vi "min data out.vi"(6 "Numeric":i32, 8 "error in (no error)":errorcluster, 9 "out time":string[](array[string]), 10 "in time":string[](array[string]), 11 "Count in":string[](array[string])) -> (0 "error out":errorcluster, 2 "string min":string[](array[string]), 3 "duration":dbl[](array[numeric]), 5 "COUNT OF ARRAY":dbl, 7 "DURATION SUM OF ARRAY":dbl)   [LabVIEW 2017]
panel:
  out "last count in min":dbl[][](array[numeric])
  out "sum":dbl
  out "Array 3":dbl[][](array[numeric])
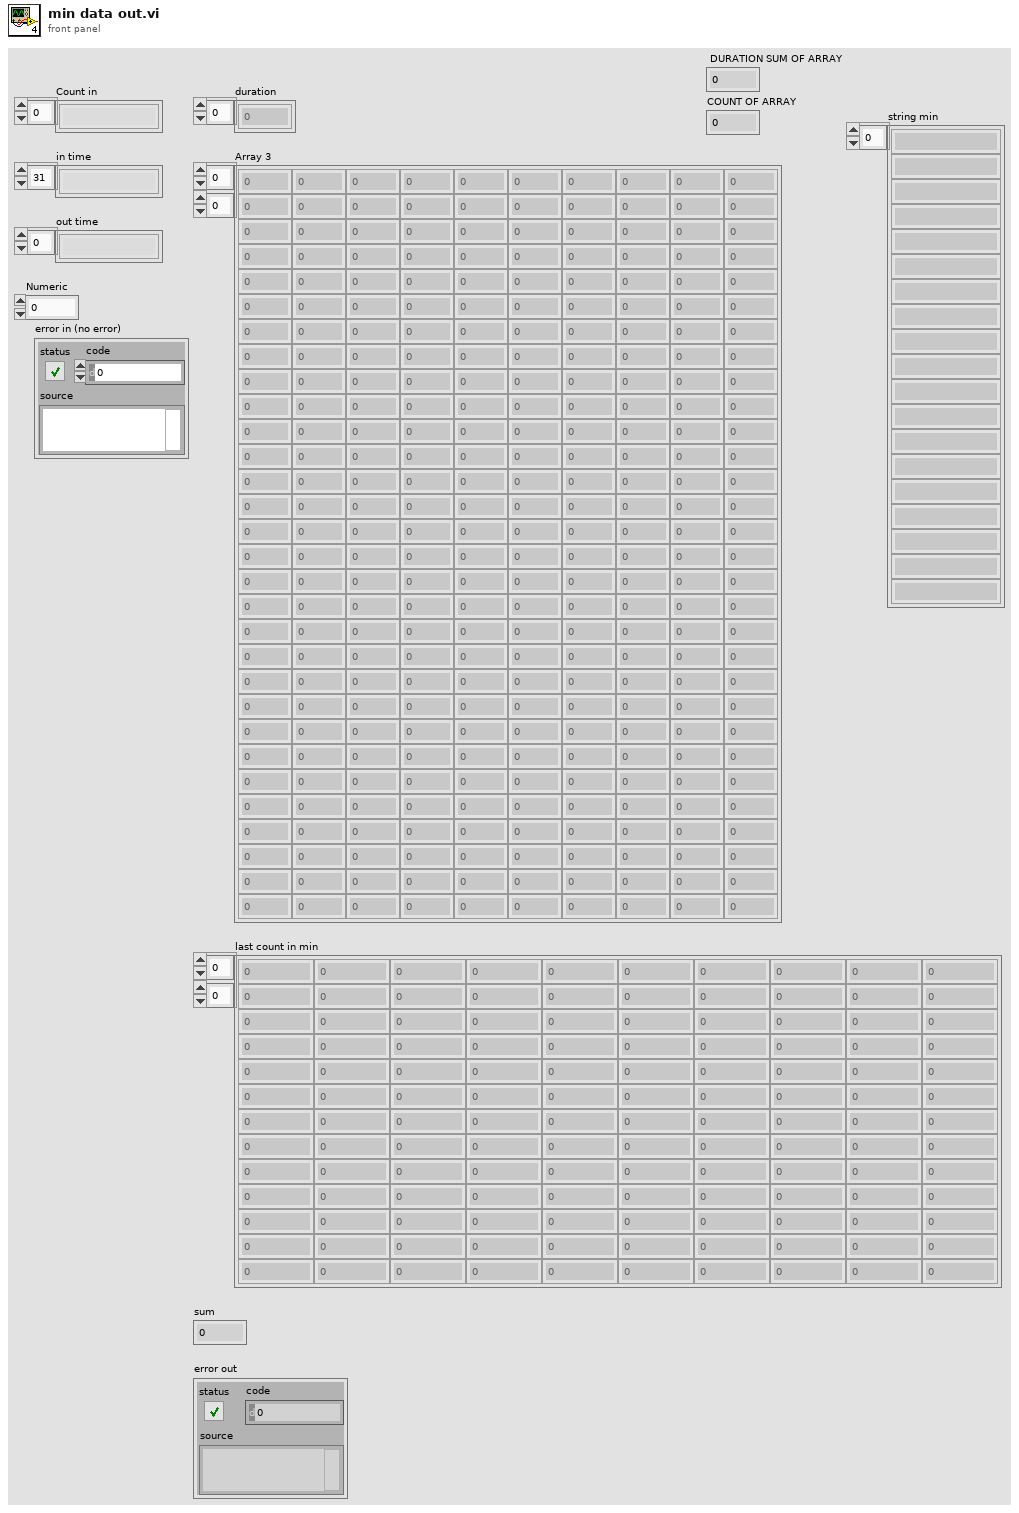
[diagram p1: front panel]
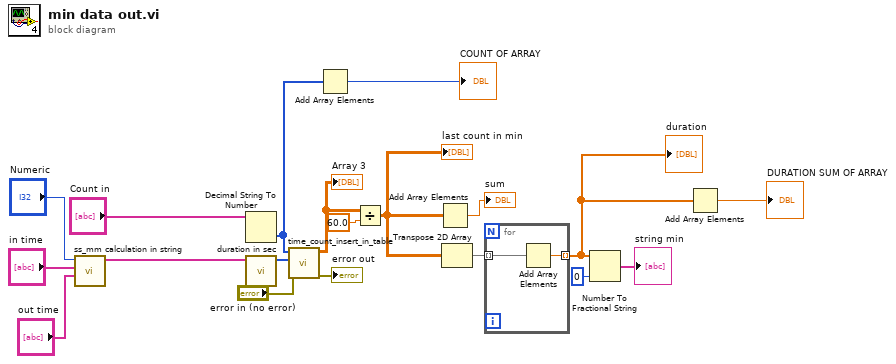
[diagram p0: block diagram]
diagram:
  n1 = call "ss_mm calculation in string.vi"("Table 2"="out time", "Table"="in time", "Numeric"="Numeric") -> ("Array 2"=w11:string[])  [unwired: 7 in, 1 out]
  n2 = Decimal String To Number(string="Count in") -> (number=w2:i32[])  [unwired: 2 in, 1 out]
  n3 = call "duration in sec.vi"("input time mm:ss"=w11) -> ("total in sec"=w17:i32[])  [unwired: 10 in]
  n4 = call "time_count_insert_in_table.vi"("error in (no error)"="error in (no error)", "time in sec"=w17, "bd count array"=w2) -> ("error out"=→"error out":errorcluster, "Array 3"=w12:dbl[][])  [unwired: 7 in]
  "Array 3" <- w12
  n5 = Add Array Elements(numeric array=w2) -> (sum=→"COUNT OF ARRAY":i32)
  n6 = Divide(x=w12, y=60.0) -> (x/y=w15:dbl[][])
  "last count in min" <- w15
  n7 = Add Array Elements(numeric array=w15) -> (sum=→"sum":dbl)
  n8 = Transpose 2D Array(2D array=w15) -> (transposed array=w16:dbl[][])
  n9 = for {
    tunnel: w16 -> [w21] mode=indexing
    tunnel: [w20] -> w4 mode=indexing
    n10 = Add Array Elements(numeric array=w21) -> (sum=w20:dbl)
  }
  "duration" <- w4
  n11 = Number To Fractional String(number=w4, precision (6)=i16 0) -> (F-format string=→"string min":string[])  [unwired: 2 in]
  n12 = Add Array Elements(numeric array=w4) -> (sum=→"DURATION SUM OF ARRAY":dbl)
